vi "SetPosition.vi"(7 "Relative?":bool, 8 "error in (no error)":errorcluster, 10 "Position":cluster{"X":sgl, "Y":sgl, "Z":sgl}, 11 "3D Object in":refnum<class "3D Object.lvclass">) -> (0 "error out":errorcluster, 3 "3D Object out":refnum<class "3D Object.lvclass">)   [LabVIEW 2015, in "3D Object.lvclass"]
uses:
  3D Object.lvclass
  3D Object.lvclass/3D Object.ctl
  <vilib>/picture/3D Picture Control/NI_3D Picture Control.lvlib
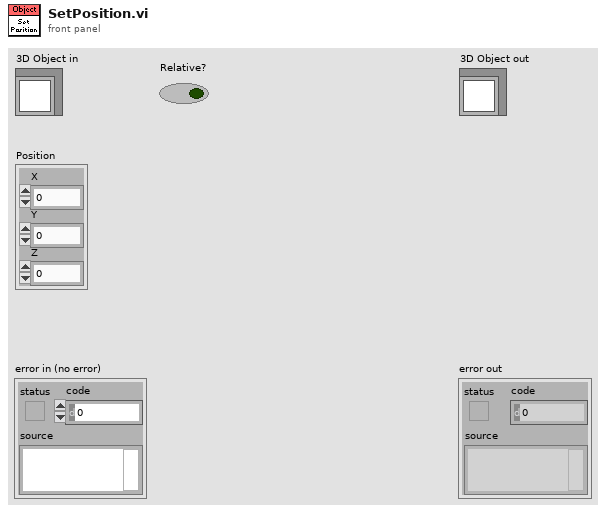
[diagram p1: front panel]
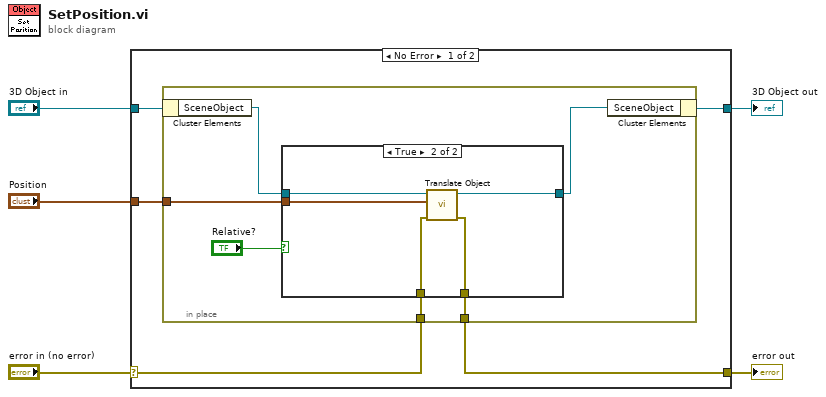
[diagram p0: block diagram]
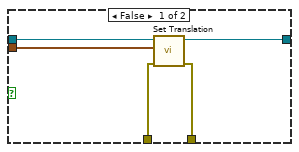
[diagram p2: hidden frame]
diagram:
  n1 = case shown="No Error" "error in (no error)" {
    selector: "error in (no error)" -> [w7 w28]
    tunnel: [w6 w28] -> w4
    tunnel: [w9 w27] -> w2
    tunnel: "3D Object in" -> [w10 w27]
    tunnel: "Position" -> [w8 _]
    frame No Error {
      n2 = in-place {
        in-place-border: w8 -> [w16]
        in-place-border: w7 -> [w13]
        in-place-border: [w12] -> w6
        n3 = in-place-cluster #1(w10) -> ("SceneObject"=w15:refnum<vi>)
        n4 = case shown="True" "Relative?" {
          tunnel: w16 -> [w21 w22]
          tunnel: w15 -> [w20 w26]
          tunnel: [w19 w25] -> w14
          tunnel: w13 -> [w18 w24]
          tunnel: [w17 w23] -> w12
          frame False {
            n5 = call <vilib>:"Set Translation.vi"("error in (no error)"=w18, "Translation"=w21, "Scene Object"=w20) -> ("error out"=w17:errorcluster, "Translated Object"=w19:refnum<vi>)  [unwired: 7 out]
          }
          frame True {
            n6 = call <vilib>:"Translate Object.vi"("error in (no error)"=w24, "Translation"=w22, "Scene.Object In"=w26) -> ("error out"=w23:errorcluster, "Scene.Object Out"=w25:refnum<vi>)  [unwired: 7 out]
          }
        }
        n7 = in-place-cluster #1("SceneObject"=w14) -> (w9:refnum<class "3D Object.lvclass">)
      }
    }
    frame Error {
    }
  }
  "error out" <- w4
  "3D Object out" <- w2
